vi "Diff_Drive_Simulated_Hardware_Simple.vi"(7 "k_magic":dbl, 8 "delta_t":dbl, 9 "b_length":dbl, 10 "%v_bus_right":dbl, 11 "%v_bus_left":dbl) -> (0 "v_angular":dbl, 1 "x_angular":dbl, 2 "a_linear":dbl, 3 "v_linear":dbl, 4 "a_angular":dbl, 5 "x_linear":dbl)   [LabVIEW 2019]
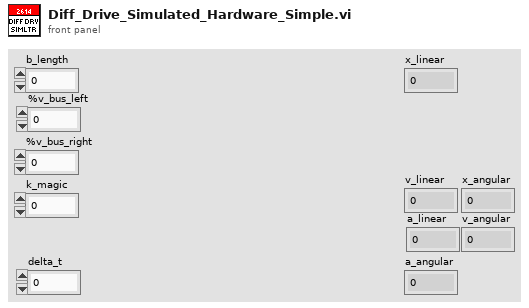
[diagram p1: front panel]
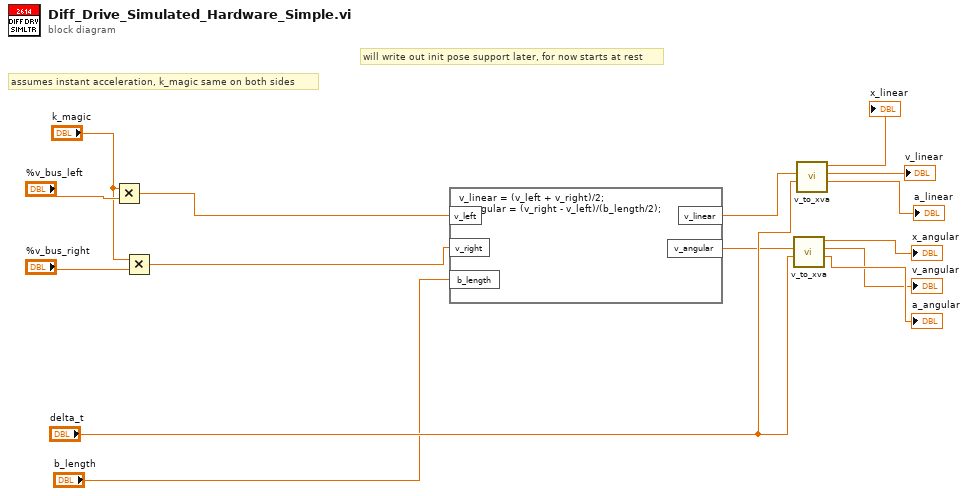
[diagram p0: block diagram]
diagram:
  # "assumes instant acceleration, k_magic same on both sides"
  # "will write out init pose support later, for now starts at rest"
  n1 = Multiply(x="k_magic", y="%v_bus_left") -> (x*y=w3:dbl)
  n2 = Multiply(x="k_magic", y="%v_bus_right") -> (x*y=w2:dbl)
  n3 = formula code="v_linear = (v_left + v_right)/2;\nv_angular = (v_right - v_left)/(b_length/2);"("v_left"=w3, "v_right"=w2, "b_length"="b_length") -> ("v_angular"=w9:dbl, "v_linear"=w8:dbl)
  n4 = call "v_to_xva.vi"("dt"="delta_t", "v"=w9) -> ("a_out"=→"a_angular":dbl, "v_out"=→"v_angular":dbl, "x_out"=→"x_angular":dbl)  [unwired: 7 in]
  n5 = call "v_to_xva.vi"("dt"="delta_t", "v"=w8) -> ("a_out"=→"a_linear":dbl, "v_out"=→"v_linear":dbl, "x_out"=→"x_linear":dbl)  [unwired: 7 in]
